vi "Get String.vi"(6 "LV Type":variant, 8 "error in (no error)":errorcluster, 9 "Data Type (default value)":string, 10 "Offset":i32, 11 "JSON":string) -> (0 "error out":errorcluster, 1 "String":string, 2 "Offset past match":i32)   [LabVIEW 2017, in "JSONtext.lvlib"]
uses:
  JSONtext.lvlib
  Unescape JSON string.vi
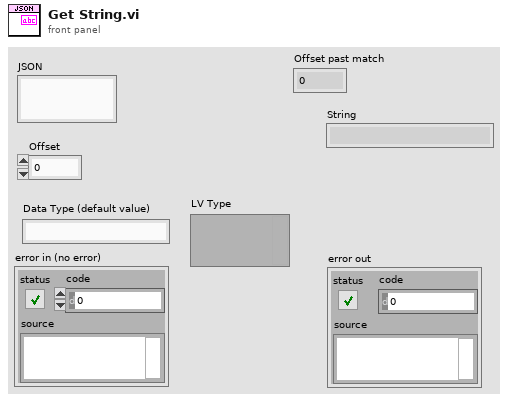
[diagram p1: front panel]
types:
  T1 = typedef "JSONtext.lvlib/Parsing State.ctl" = enum16{"Parser Error", "Object", "Array", "String", "Number/Other", "Leading Whitespace", "Object end", "Array end", "Value end"}
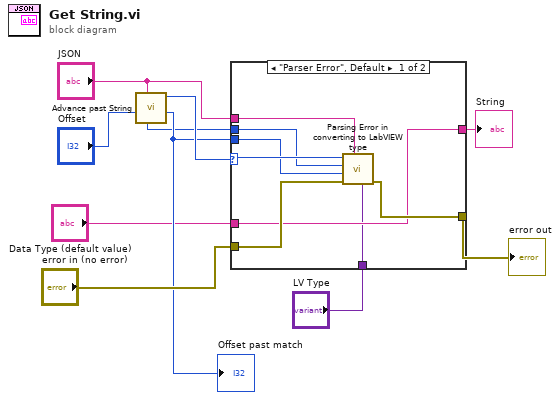
[diagram p0: block diagram]
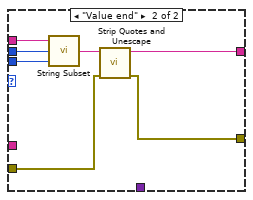
[diagram p2: hidden frame]
diagram:
  n1 = call "Advance past String.vi"("JSON"="JSON", "Offset"="Offset") -> ("Offset past match"=w4:i32, "State"=w8:T1, "Value start out"=w3:i32)  [unwired: 7 in]
  "Offset past match" <- w4
  n2 = case shown="\"Parser Error\", Default" w8 {
    selector: w8 -> [w16 _]
    tunnel: "JSON" -> [w13 w24]
    tunnel: [w18 w22] -> w7
    tunnel: "error in (no error)" -> [w17 w23]
    tunnel: [w12 w21] -> w5
    tunnel: w3 -> [w15 w20]
    tunnel: w4 -> [w14 w19]
    tunnel: "Data Type (default value)" -> [w12 _]
    tunnel: "LV Type" -> [w11 _]
    frame "Parser Error", Default {
      n3 = call "Parsing Error in converting to LabVIEW type.vi"("LV Type"=w11, "JSON"=w13, "error in (no error)"=w17, "Offset past match"=w14, "Value start"=w15, "State"=w16) -> ("error out"=w18:errorcluster)  [unwired: 5 in]
    }
    frame "Value end" {
      n4 = call "String Subset.vi"("Offset past End"=w19, "Start offset"=w20, "JSON"=w24) -> ("substring"=w25:string)  [unwired: 2 in]
      n5 = call "Strip Quotes and Unescape.vi"("error in (no error)"=w23, "String"=w25) -> ("error out"=w22:errorcluster, "result string"=w21:string)  [unwired: 8 in]
    }
  }
  "error out" <- w7
  "String" <- w5
